vi "Weighted_Fast_Response_Stats_1.vi"(0 "U":dbl[](array[numeric]) format="%.2f", 5 "Weighting":dbl[](array[numeric]) format="%.2f", 9 "Use Weighting?":bool, 11 "Shift in":dbl[](array[numeric]) format="%.2f", 12 "Block No":i32=1) -> (2 "U":dbl, 3 "u^2":dbl, 4 "u^3":dbl, 6 "u^4":dbl, 8 "Skew":dbl, 10 "Kurt":dbl, 14 "% u'/U":dbl, 15 "Shift out":dbl[](array[numeric]) format="%.2f")   [LabVIEW 2011]
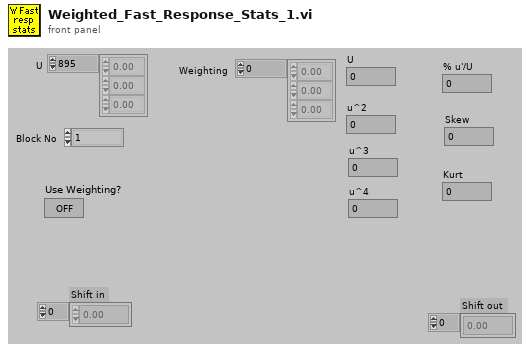
[diagram p1: front panel]
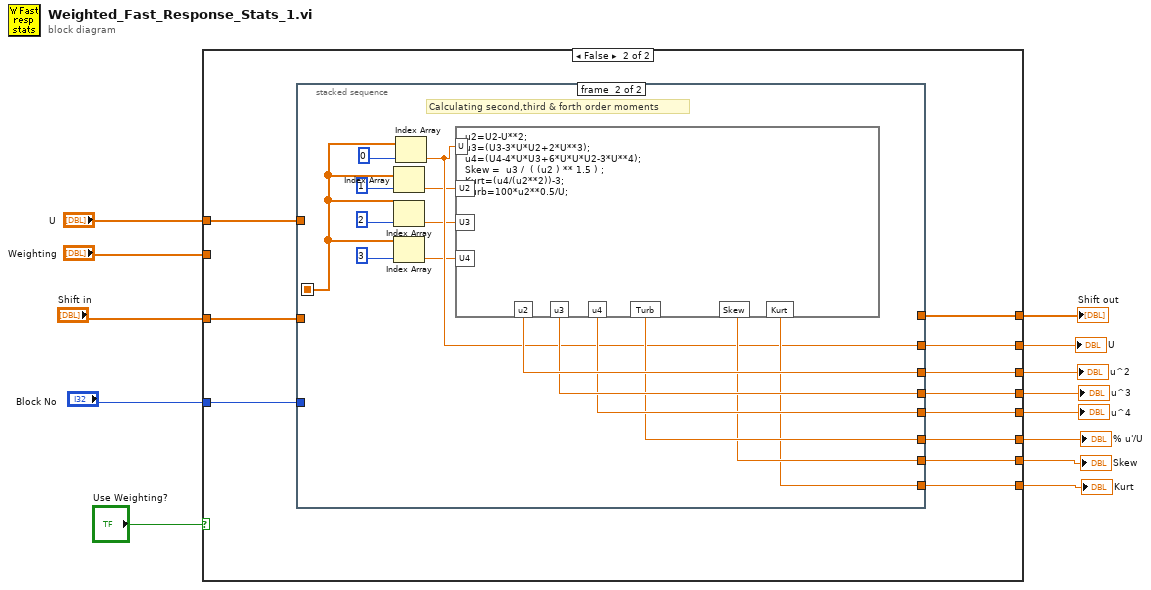
[diagram p0: block diagram]
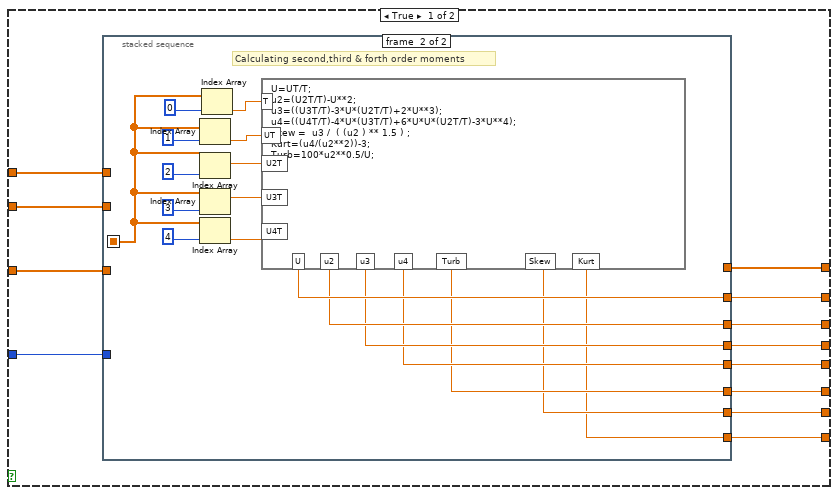
[diagram p2: hidden frame]
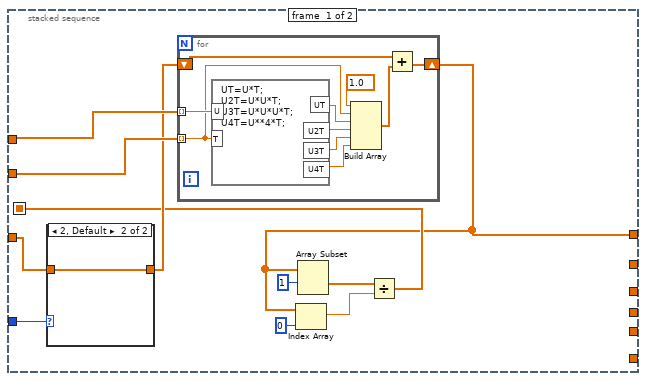
[diagram p3: hidden frame]
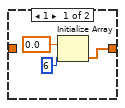
[diagram p4: hidden frame]
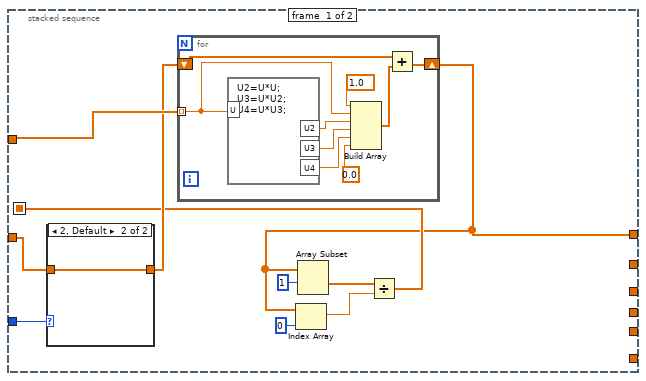
[diagram p5: hidden frame]
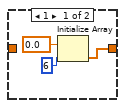
[diagram p6: hidden frame]
diagram:
  n1 = case shown="False" "Use Weighting?" {
    tunnel: "Shift in" -> [w25 w79]
    tunnel: [w24 w78] -> w12
    tunnel: "U" -> [w23 w77]
    tunnel: "Weighting" -> [w22 _]
    tunnel: "Block No" -> [w21 w76]
    tunnel: [w20 w75] -> w8
    tunnel: [w19 w74] -> w7
    tunnel: [w18 w73] -> w6
    tunnel: [w17 w72] -> w5
    tunnel: [w16 w71] -> w4
    tunnel: [w15 w70] -> w3
    tunnel: [w14 w69] -> w2
    frame True {
      n2 = stacked-sequence {
        seq-local: [w27 _] -> [_ w65]
        tunnel: w23 -> [w36 _]
        tunnel: [w26 _] -> w24
        tunnel: w25 -> [w29 _]
        tunnel: w22 -> [w35 _]
        tunnel: w21 -> [w30 _]
        tunnel: [_ w57] -> w20
        tunnel: [_ w56] -> w19
        tunnel: [_ w55] -> w18
        tunnel: [_ w54] -> w17
        tunnel: [_ w53] -> w16
        tunnel: [_ w52] -> w15
        tunnel: [_ w51] -> w14
        frame #0 {
          n3 = case shown="2, Default" w30 {
            tunnel: [w37 w40] -> w28
            tunnel: w29 -> [_ w40]
            frame 1 {
              n4 = Initialize Array(0.0 ("Element Data"), 6 ("Dimension Size")) -> (w37:dbl[])
            }
            frame 2, Default {
            }
          }
          n5 = for {
            shift-right: [w49] -> w26
            shift-left: w28 -> [w50]
            tunnel: w36 -> [w47] mode=indexing
            tunnel: w35 -> [w46] mode=indexing
            n6 = formula code="UT=U*T;\nU2T=U*U*T;\nU3T=U*U*U*T;\nU4T=U**4*T;"("U"=w47, "T"=w46) -> ("U2T"=w44:dbl, "UT"=w45:dbl, "U3T"=w43:dbl, "U4T"=w42:dbl)
            n7 = Build Array(1.0 ("Input Element"), w46, w45, w44, w43, w42) -> (w48:dbl[])
            n8 = Add(x=w50, y=w48) -> (x+y=w49:dbl[])
          }
          n9 = Index Array(array=w26, index=0 ("Index")) -> (element=w31:dbl)
          n10 = Array Subset(array=w26, index=1 ("Array Index")) -> (w32:dbl[])  [unwired: 1 in]
          n11 = Divide(x=w32, y=w31) -> (x/y=w27:dbl[])
        }
        frame #1 {
          # "Calculating second,third & forth order moments"
          n12 = Index Array(array=w65, index=1) -> (element=w61:dbl)
          n13 = Index Array(array=w65, index=2) -> (element=w60:dbl)
          n14 = Index Array(array=w65, index=3) -> (element=w59:dbl)
          n15 = Index Array(array=w65, index=4) -> (element=w58:dbl)
          n16 = Index Array(array=w65, index=0) -> (element=w62:dbl)
          n17 = formula code="U=UT/T;\nu2=(U2T/T)-U**2;\nu3=((U3T/T)-3*U*(U2T/T)+2*U**3);\nu4=((U4T/T)-4*U*(U3T/T)+6*U*U*(U2T/T)-3*U**4);\nSkew =  u3 /  ( (u2 ) ** 1.5 ) ;\nKurt=(u4/(u2**2))-3;\nTurb=100*u2**0.5/U;"("T"=w62, "UT"=w61, "U2T"=w60, "U3T"=w59, "U4T"=w58) -> ("Kurt"=w51:dbl, "Skew"=w52:dbl, "U"=w57:dbl, "u2"=w56:dbl, "u3"=w55:dbl, "u4"=w54:dbl, "Turb"=w53:dbl)
        }
      }
    }
    frame False {
      n18 = stacked-sequence {
        seq-local: [w81 _] -> [_ w115]
        tunnel: w77 -> [w89 _]
        tunnel: [w80 _] -> w78
        tunnel: w79 -> [w83 _]
        tunnel: w76 -> [w84 _]
        tunnel: [_ w106] -> w75
        tunnel: [_ w112] -> w74
        tunnel: [_ w111] -> w73
        tunnel: [_ w110] -> w72
        tunnel: [_ w109] -> w71
        tunnel: [_ w108] -> w70
        tunnel: [_ w107] -> w69
        frame #0 {
          n19 = case shown="2, Default" w84 {
            tunnel: [w90 w93] -> w82
            tunnel: w83 -> [_ w93]
            frame 1 {
              n20 = Initialize Array(0.0 ("Element Data"), 6 ("Dimension Size")) -> (w90:dbl[])
            }
            frame 2, Default {
            }
          }
          n21 = for {
            shift-right: [w101] -> w80
            shift-left: w82 -> [w102]
            tunnel: w89 -> [w98] mode=indexing
            n22 = formula code="U2=U*U;\nU3=U*U2;\nU4=U*U3;"("U"=w98) -> ("U2"=w97:dbl, "U3"=w96:dbl, "U4"=w95:dbl)
            n23 = Build Array(1.0 ("Input Element"), w98, w97, w96, w95, 0.0 ("element")) -> (w100:dbl[])
            n24 = Add(x=w102, y=w100) -> (x+y=w101:dbl[])
          }
          n25 = Index Array(array=w80, index=0 ("Index")) -> (element=w85:dbl)
          n26 = Array Subset(array=w80, index=1 ("Array Index")) -> (w86:dbl[])  [unwired: 1 in]
          n27 = Divide(x=w86, y=w85) -> (x/y=w81:dbl[])
        }
        frame #1 {
          # "Calculating second,third & forth order moments"
          n28 = Index Array(array=w115, index=1) -> (element=w105:dbl)
          n29 = Index Array(array=w115, index=2) -> (element=w104:dbl)
          n30 = Index Array(array=w115, index=3) -> (element=w103:dbl)
          n31 = Index Array(array=w115, index=0) -> (element=w106:dbl)
          n32 = formula code="u2=U2-U**2;\nu3=(U3-3*U*U2+2*U**3);\nu4=(U4-4*U*U3+6*U*U*U2-3*U**4);\nSkew =  u3 /  ( (u2 ) ** 1.5 ) ;\nKurt=(u4/(u2**2))-3;\nTurb=100*u2**0.5/U;"("U"=w106, "U2"=w105, "U3"=w104, "U4"=w103) -> ("Kurt"=w107:dbl, "Skew"=w108:dbl, "u2"=w112:dbl, "u3"=w111:dbl, "u4"=w110:dbl, "Turb"=w109:dbl)
        }
      }
    }
  }
  "Shift out" <- w12
  "U" <- w8
  "u^2" <- w7
  "u^3" <- w6
  "u^4" <- w5
  "% u'/U" <- w4
  "Skew" <- w3
  "Kurt" <- w2
